vi "Get Internal Data Info.vi"(8 "error in (no error)":errorcluster, 11 "CSM-Helper in":refnum<class "CSM-Helper.lvclass">) -> (0 "error out":errorcluster, 2 "Array":cluster{"Data":string, "prototype":variant}[](array[cluster]), 3 "CSM-Helper out":refnum<class "CSM-Helper.lvclass">)   [LabVIEW 2020, in "CSM-Helper.lvclass"]
uses:
  CSM-Helper.lvclass
  CSM-Helper.lvclass/CSM-Helper.ctl
  <userlib>/_NEVSTOP/Communicable State Machine(CSM)/addons/API-String-Arugments-Support/API String Arguments Support.lvlib
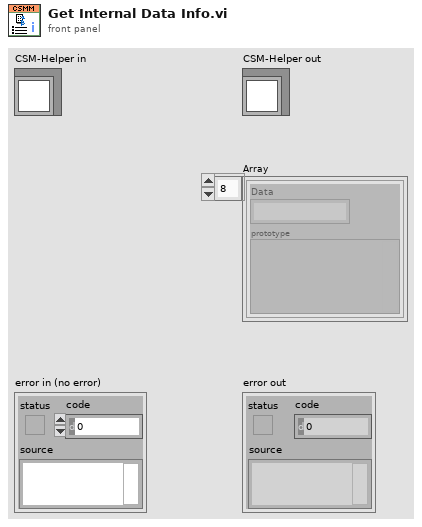
[diagram p1: front panel]
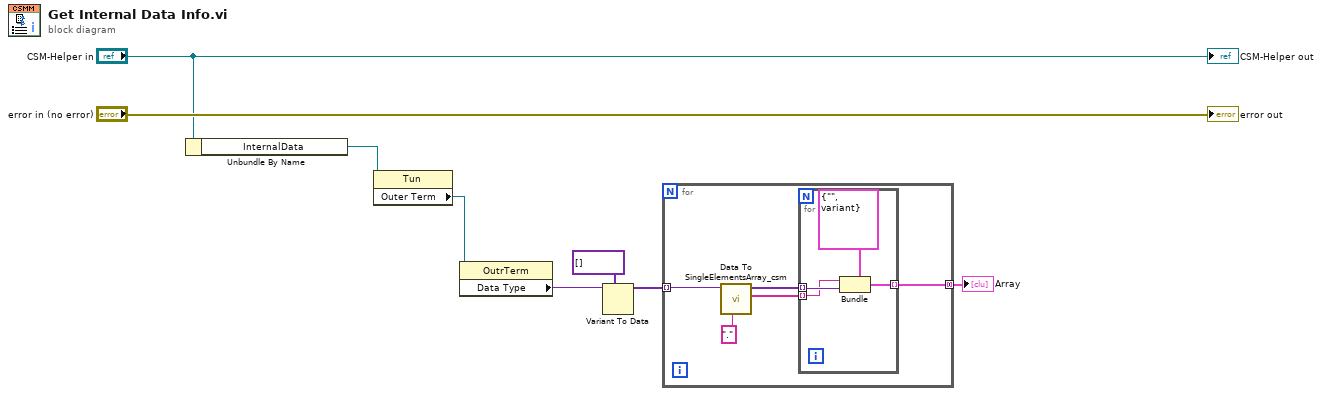
[diagram p0: block diagram]
diagram:
  n1 = Unbundle By Name("CSM-Helper in") -> ("InternalData"=w6:refnum<vi>)
  n2 = property class="Tun"(reference=w6) -> ("Outer Term"=w5:refnum<vi>)  [unwired: 1 in, 2 out]
  n3 = property class="OutrTerm"(reference=w5) -> ("Data Type"=w2:variant)  [unwired: 1 in, 2 out]
  n4 = Variant To Data(type=variant[] [] ("Array"), Variant=w2) -> (data=w3:variant[])  [unwired: 1 in, 1 out]
  n5 = for {
    tunnel: w3 -> [w12] mode=indexing
    tunnel: [w9] -> w1 mode=concatenating
    n6 = call <userlib>:"Data To SingleElementsArray_csm.vi"("Seperator(/)"=".", "Cluster"=w12) -> ("Full NameList"=w10:string[], "DataElementArray"=w11:variant[])  [unwired: 7 in, 1 out]
    n7 = for {
      tunnel: w11 -> [w17] mode=indexing
      tunnel: w10 -> [w16] mode=indexing
      tunnel: [w14] -> w9 mode=indexing
      n8 = Bundle(cluster=cluster{"Data":string, "prototype":variant} {"Data"="", "prototype"=variant}, "Data"=w16, "prototype"=w17) -> (w14:cluster{"Data":string, "prototype":variant})
    }
  }
  "Array" <- w1
  "error out" <- "error in (no error)"
  "CSM-Helper out" <- "CSM-Helper in"
